vi "shooter_begin.vi"() -> ()   [LabVIEW 2012]
uses:
  <vilib>/Rock Robotics/WPI/CAN/Jaguar/SubVIs/WPI_CANJaguar_BrakeCoastMode.ctl
  <vilib>/Rock Robotics/WPI/CAN/Jaguar/SubVIs/WPI_CANJaguar_ControlMode.ctl
  <vilib>/Rock Robotics/SystemInterfaces/Typedef/FPGA_TypedefAnalogModule.ctl
  <vilib>/Rock Robotics/SystemInterfaces/AI/FPGA_AIChannel.ctl
  <vilib>/Rock Robotics/WPI/CAN/Jaguar/SubVIs/WPI_CANJaguar_SpeedReference.ctl
  <vilib>/Rock Robotics/WPI/MotorControl/WPI_MotorControlOpenCANJaguar.vi
panel:
  out "error out":errorcluster
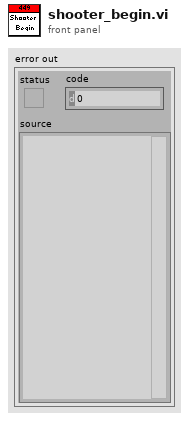
[diagram p1: front panel]
types:
  T1 = typedef "FPGA_AIChannel.ctl" = enum8{"AI 1", "AI 2", "AI 3", "AI 4", "AI 5", "AI 6", "AI 7", "AI 8", "Invalid"}
  T2 = typedef "FPGA_TypedefAnalogModule.ctl" = enum16{"Analog Module 1", "Analog Module 2"}
  T3 = typedef "WPI_CANJaguar_BrakeCoastMode.ctl" = enum8{"Jumper", "Brake", "Coast"}
  T4 = typedef "WPI_CANJaguar_ControlMode.ctl" = enum8{"Percent VBus", "Current", "Speed", "Position", "Voltage"}
  T5 = typedef "WPI_AnalogChannelDevRef.ctl" = cluster{"DevStatus":errorcluster, "Analog Module":T2, "Analog Channel":T1}
  T6 = typedef "WPI_MotorControlDeviceRef.ctl" = cluster{"DeviceStatus":errorcluster, "Type":enum16{"PWM", "CAN"}, "PWM":cluster{"Digital Module":T7, "PWM Channel":T8, "DeadBand":T9}, "CAN":cluster{"Device Number":u8, "Control Mode":T4, "Semaphore":T10, "Max Vout":dbl}, "Invert":bool, "TransformRef":T11, "InvTransformRef":T11}
  T7 = typedef "FPGA_TypedefDigitalModule.ctl" = enum16{"Digital Module 1", "Digital Module 2"}
  T8 = typedef "FPGA_DIOPWMChannel.ctl" = enum8{"PWM 1", "PWM 2", "PWM 3", "PWM 4", "PWM 5", "PWM 6", "PWM 7", "PWM 8", "PWM 9", "PWM 10", "Invalid"}
  T9 = typedef "WPI_PWMDeadband.ctl" = cluster{"Name":string, "maxPositivePwm":i32, "minPositivePwm":i32, "centerPwm":i32, "maxNegativePwm":i32, "minNegativePwm":i32, "angularRange":u16}
  T10 = typedef "Semaphore RefNum" = refnum<k1>
  T11 = typedef "WPI_PWMTransform_ConPane.ctl" = refnum<vi>
  T12 = typedef "WPI_CANJaguar_SpeedReference.ctl" = u8
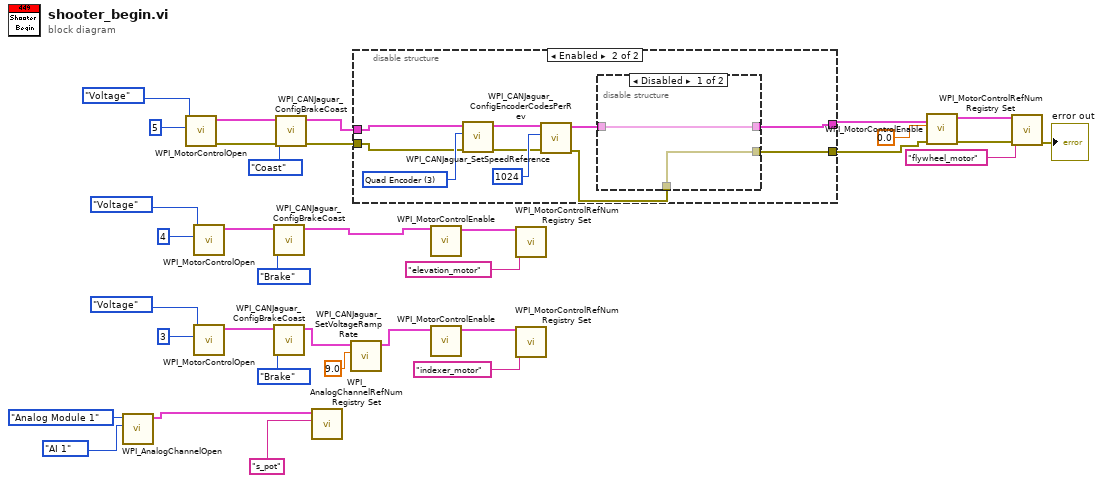
[diagram p0: block diagram]
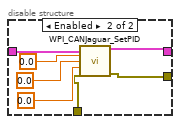
[diagram p3: hidden frame]
diagram:
  n1 = call <vilib>:"WPI_AnalogChannelOpen.vi"("Analog Channel"=FPGA_AIChannel."AI 1", "Analog Module (Module 1)"=FPGA_TypedefAnalogModule."Analog Module 1") -> ("AIDeviceRef"=w12:T5)  [unwired: 8 in, 1 out]
  n2 = call-poly <vilib>:"WPI_MotorControlOpen.vi"("Device Number"=u8 5, "Control Mode"=WPI_CANJaguar_ControlMode."Voltage") -> ("error out"=w5:errorcluster, "MotorControlDeviceRef"=w34:T6)  [unwired: 8 in]
  n3 = call-poly <vilib>:"WPI_MotorControlOpen.vi"("Device Number"=u8 4, "Control Mode"=WPI_CANJaguar_ControlMode."Voltage") -> ("MotorControlDeviceRef"=w28:T6)  [unwired: 8 in, 1 out]
  n4 = call-poly <vilib>:"WPI_MotorControlOpen.vi"("Device Number"=u8 3, "Control Mode"=WPI_CANJaguar_ControlMode."Voltage") -> ("MotorControlDeviceRef"=w21:T6)  [unwired: 8 in, 1 out]
  n5 = call <vilib>:"WPI_CANJaguar_ConfigBrakeCoast.vi"("Brake / Coast Mode"=WPI_CANJaguar_BrakeCoastMode."Brake", "CAN Jaguar Ref"=w28) -> ("CAN Jaguar Ref Out"=w25:T6)  [unwired: 8 in, 1 out]
  n6 = call <vilib>:"WPI_CANJaguar_ConfigBrakeCoast.vi"("Brake / Coast Mode"=WPI_CANJaguar_BrakeCoastMode."Brake", "CAN Jaguar Ref"=w21) -> ("CAN Jaguar Ref Out"=w15:T6)  [unwired: 8 in, 1 out]
  n7 = call <vilib>:"WPI_CANJaguar_ConfigBrakeCoast.vi"("error in (no error)"=w5, "Brake / Coast Mode"=WPI_CANJaguar_BrakeCoastMode."Coast", "CAN Jaguar Ref"=w34) -> ("error out"=w4:errorcluster, "CAN Jaguar Ref Out"=w8:T6)  [unwired: 7 in]
  n8 = call <vilib>:"WPI_AnalogChannelRefNum Registry Set.vi"("refnum name"="s_pot", "AIDeviceRef"=w12) -> ()  [unwired: 8 in, 2 out]
  n9 = call <vilib>:"WPI_CANJaguar_SetVoltageRampRate.vi"("VoltageRampRate (V/s)"=9.0, "CAN Jaguar Ref"=w15) -> ("CAN Jaguar Ref Out"=w14:T6)  [unwired: 8 in, 1 out]
  n10 = disable-structure shown="Enabled" {
    disable-tunnel: w8 -> [w36 w44]
    disable-tunnel: [w36 w41] -> w6
    disable-tunnel: w4 -> [w35 w39]
    disable-tunnel: [w35 w37] -> w3
    frame Disabled {
    }
    frame Enabled {
      w46 = T12 3 items=["Encoder"=0, "Inv Encoder"=2, "Quad Encoder"=3, "None"=255] ("Speed Reference")
      n11 = call <vilib>:"WPI_CANJaguar_SetSpeedReference.vi"("error in (no error)"=w39, "Speed Reference"=w46, "CAN Jaguar Ref"=w44) -> ("error out"=w40:errorcluster, "CAN Jaguar Ref Out"=w45:T6)  [unwired: 7 in]
      n12 = call <vilib>:"WPI_CANJaguar_ConfigEncoderCodesPerRev.vi"("error in (no error)"=w40, "Encoder Codes Per Rev"=u16 1024, "CAN Jaguar Ref"=w45) -> ("error out"=w38:errorcluster, "CAN Jaguar Ref Out"=w42:T6)  [unwired: 7 in]
      n13 = disable-structure shown="Disabled" {
        disable-tunnel: w42 -> [w48 w55]
        disable-tunnel: [w48 w54] -> w41
        disable-tunnel: w38 -> [w47 w50]
        disable-tunnel: [w47 w49] -> w37
        frame Disabled {
        }
        frame Enabled {
          n14 = call <vilib>:"WPI_CANJaguar_SetPID.vi"("CAN Jaguar Ref"=w55, "P"=0.0, "I"=0.0, "D"=0.0, "error in (no error)"=w50) -> ("CAN Jaguar Ref Out"=w54:T6, "error out"=w49:errorcluster)  [unwired: 9 in]
        }
      }
    }
  }
  n15 = call <vilib>:"WPI_MotorControlEnable.vi"("CAN Jaguar Ref"=w25) -> ("CAN Jaguar Ref Out"=w27:T6)  [unwired: 9 in, 1 out]
  n16 = call <vilib>:"WPI_MotorControlEnable.vi"("CAN Jaguar Ref"=w14) -> ("CAN Jaguar Ref Out"=w20:T6)  [unwired: 9 in, 1 out]
  n17 = call <vilib>:"WPI_MotorControlRefNum Registry Set.vi"("refnum name"="elevation_motor", "MotorControlDevRef"=w27) -> ()  [unwired: 8 in, 2 out]
  n18 = call <vilib>:"WPI_MotorControlRefNum Registry Set.vi"("refnum name"="indexer_motor", "MotorControlDevRef"=w20) -> ()  [unwired: 8 in, 2 out]
  n19 = call <vilib>:"WPI_MotorControlEnable.vi"("error in (no error)"=w3, "Encoder Initial Position"=0.0, "CAN Jaguar Ref"=w6) -> ("error out"=w2:errorcluster, "CAN Jaguar Ref Out"=w33:T6)  [unwired: 7 in]
  n20 = call <vilib>:"WPI_MotorControlRefNum Registry Set.vi"("error in (no error)"=w2, "refnum name"="flywheel_motor", "MotorControlDevRef"=w33) -> ("error out"=→"error out":errorcluster)  [unwired: 7 in, 1 out]
